vi "ASIC_THx MITAD RANGO.vi"(7 "Espera acceso USB":u32, 8 "error in":errorcluster, 10 "Canal":u8, 11 "ftHandle_in":u32) -> (0 "error out":errorcluster, 3 "ftHandle_out":u32)   [LabVIEW 2009]
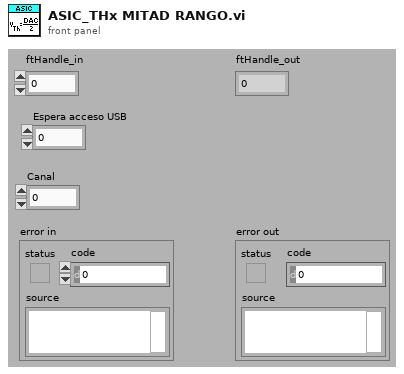
[diagram p1: front panel]
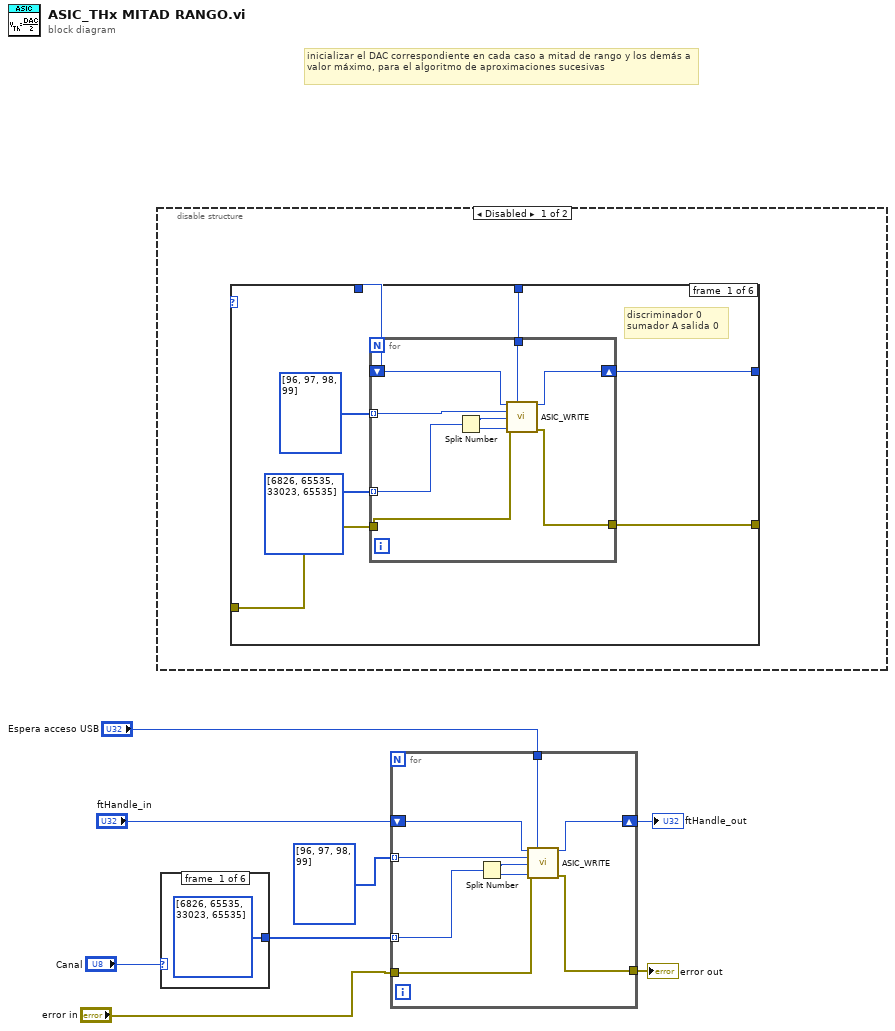
[diagram p0: block diagram]
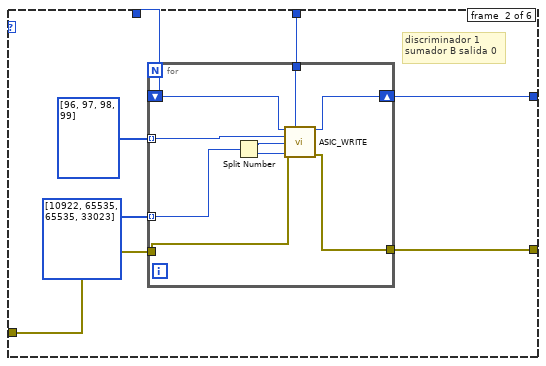
[diagram p2: hidden frame]
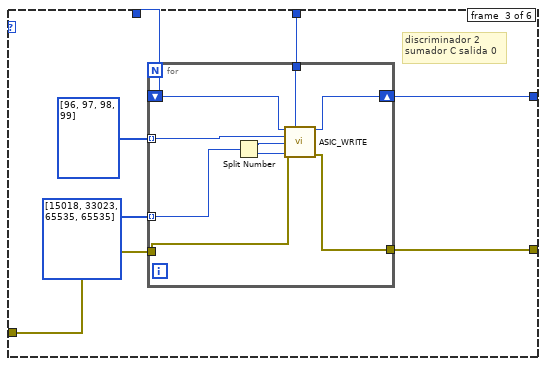
[diagram p3: hidden frame]
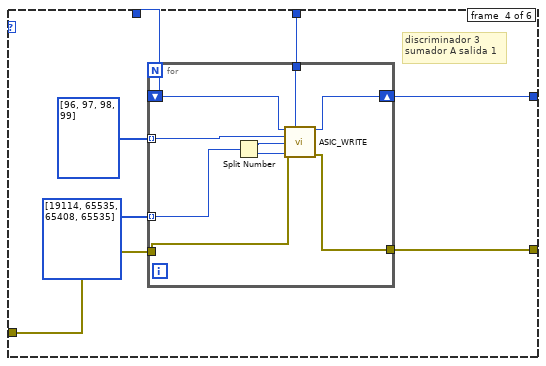
[diagram p4: hidden frame]
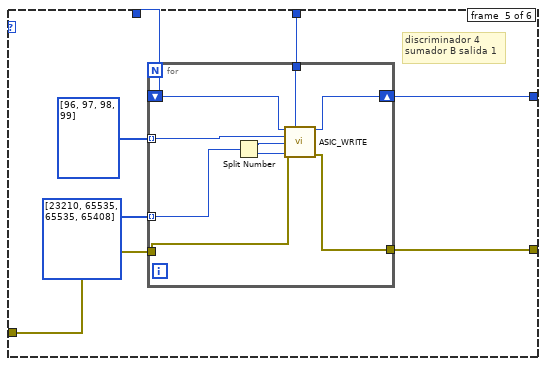
[diagram p5: hidden frame]
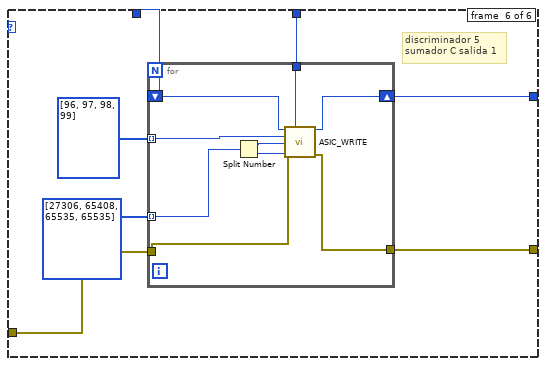
[diagram p6: hidden frame]
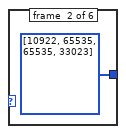
[diagram p8: hidden frame]
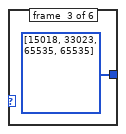
[diagram p9: hidden frame]
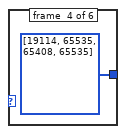
[diagram p10: hidden frame]
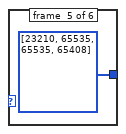
[diagram p11: hidden frame]
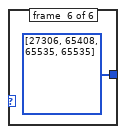
[diagram p12: hidden frame]
diagram:
  # "inicializar el DAC correspondiente en cada caso a mitad de rango y los demás a valor máximo, para el algoritmo de aproximaciones sucesivas"
  n1 = disable-structure shown="Disabled" {
    frame #0 {
      n2 = case shown="5.." {
        tunnel: [w15 w31 w47 w63 w79 w95] -> w10
        tunnel: _ -> [w14 w30 w46 w62 w78 w94]
        tunnel: [w13 w29 w45 w61 w77 w93] -> _
        tunnel: [w12 w27 w44 w60 w76 w92] -> _
        tunnel: [w11 w28 w43 w59 w75 w91] -> w9
        selector: _ -> [_ _ _ _ _ _]
        frame #0 {
          # "discriminador 0\nsumador A salida 0"
          n3 = for {
            shift-right: [w25] -> w12
            shift-left: w15 -> [w26]
            tunnel: i32[] [96, 97, 98, 99] -> [w24] mode=indexing
            tunnel: u16[] [6826, 65535, 33023, 65535] -> [w18] mode=indexing
            tunnel: w14 -> [w23]
            tunnel: [w22] -> w13
            tunnel: w11 -> [w21]
            n4 = Split Number(x=w18) -> (hi(x)=w20:u8, lo(x)=w19:u8)
            n5 = call "ASIC_WRITE.vi"("ftHandle_in"=w26, "Espera acceso USB"=w21, "Direccion Registro Asic"=w24, "Byte Alto"=w20, "Byte Bajo"=w19, "error in"=w23) -> ("ftHandle_out"=w25:u32, "error out"=w22:errorcluster)  [unwired: 8 in]
          }
        }
        frame #1 {
          # "discriminador 1\nsumador B salida 0"
          n6 = for {
            shift-right: [w41] -> w27
            shift-left: w31 -> [w42]
            tunnel: i32[] [96, 97, 98, 99] -> [w40] mode=indexing
            tunnel: u16[] [10922, 65535, 65535, 33023] -> [w34] mode=indexing
            tunnel: w30 -> [w39]
            tunnel: [w38] -> w29
            tunnel: w28 -> [w37]
            n7 = Split Number(x=w34) -> (hi(x)=w36:u8, lo(x)=w35:u8)
            n8 = call "ASIC_WRITE.vi"("ftHandle_in"=w42, "Espera acceso USB"=w37, "Direccion Registro Asic"=w40, "Byte Alto"=w36, "Byte Bajo"=w35, "error in"=w39) -> ("ftHandle_out"=w41:u32, "error out"=w38:errorcluster)  [unwired: 8 in]
          }
        }
        frame #2 {
          # "discriminador 2\nsumador C salida 0"
          n9 = for {
            shift-right: [w57] -> w44
            shift-left: w47 -> [w58]
            tunnel: i32[] [96, 97, 98, 99] -> [w56] mode=indexing
            tunnel: u16[] [15018, 33023, 65535, 65535] -> [w50] mode=indexing
            tunnel: w46 -> [w55]
            tunnel: [w54] -> w45
            tunnel: w43 -> [w53]
            n10 = Split Number(x=w50) -> (hi(x)=w52:u8, lo(x)=w51:u8)
            n11 = call "ASIC_WRITE.vi"("ftHandle_in"=w58, "Espera acceso USB"=w53, "Direccion Registro Asic"=w56, "Byte Alto"=w52, "Byte Bajo"=w51, "error in"=w55) -> ("ftHandle_out"=w57:u32, "error out"=w54:errorcluster)  [unwired: 8 in]
          }
        }
        frame #3 {
          # "discriminador 3\nsumador A salida 1"
          n12 = for {
            shift-right: [w73] -> w60
            shift-left: w63 -> [w74]
            tunnel: i32[] [96, 97, 98, 99] -> [w72] mode=indexing
            tunnel: u16[] [19114, 65535, 65408, 65535] -> [w66] mode=indexing
            tunnel: w62 -> [w71]
            tunnel: [w70] -> w61
            tunnel: w59 -> [w69]
            n13 = Split Number(x=w66) -> (hi(x)=w68:u8, lo(x)=w67:u8)
            n14 = call "ASIC_WRITE.vi"("ftHandle_in"=w74, "Espera acceso USB"=w69, "Direccion Registro Asic"=w72, "Byte Alto"=w68, "Byte Bajo"=w67, "error in"=w71) -> ("ftHandle_out"=w73:u32, "error out"=w70:errorcluster)  [unwired: 8 in]
          }
        }
        frame #4 {
          # "discriminador 4\nsumador B salida 1"
          n15 = for {
            shift-right: [w89] -> w76
            shift-left: w79 -> [w90]
            tunnel: i32[] [96, 97, 98, 99] -> [w88] mode=indexing
            tunnel: u16[] [23210, 65535, 65535, 65408] -> [w82] mode=indexing
            tunnel: w78 -> [w87]
            tunnel: [w86] -> w77
            tunnel: w75 -> [w85]
            n16 = Split Number(x=w82) -> (hi(x)=w84:u8, lo(x)=w83:u8)
            n17 = call "ASIC_WRITE.vi"("ftHandle_in"=w90, "Espera acceso USB"=w85, "Direccion Registro Asic"=w88, "Byte Alto"=w84, "Byte Bajo"=w83, "error in"=w87) -> ("ftHandle_out"=w89:u32, "error out"=w86:errorcluster)  [unwired: 8 in]
          }
        }
        frame #5 {
          # "discriminador 5\nsumador C salida 1"
          n18 = for {
            shift-right: [w105] -> w92
            shift-left: w95 -> [w106]
            tunnel: i32[] [96, 97, 98, 99] -> [w104] mode=indexing
            tunnel: u16[] [27306, 65408, 65535, 65535] -> [w98] mode=indexing
            tunnel: w94 -> [w103]
            tunnel: [w102] -> w93
            tunnel: w91 -> [w101]
            n19 = Split Number(x=w98) -> (hi(x)=w100:u8, lo(x)=w99:u8)
            n20 = call "ASIC_WRITE.vi"("ftHandle_in"=w106, "Espera acceso USB"=w101, "Direccion Registro Asic"=w104, "Byte Alto"=w100, "Byte Bajo"=w99, "error in"=w103) -> ("ftHandle_out"=w105:u32, "error out"=w102:errorcluster)  [unwired: 8 in]
          }
        }
      }
    }
    frame #1 {
    }
  }
  n21 = case shown="0, Default" "Canal" {
    tunnel: [u16[] [6826, 65535, 33023, 65535] u16[] [10922, 65535, 65535, 33023] u16[] [15018, 33023, 65535, 65535] u16[] [19114, 65535, 65408, 65535] u16[] [23210, 65535, 65535, 65408] u16[] [27306, 65408, 65535, 65535]] -> w6
    frame #0 {
    }
    frame #1 {
    }
    frame #2 {
    }
    frame #3 {
    }
    frame #4 {
    }
    frame #5 {
    }
  }
  n22 = for {
    shift-right: [w120] -> w2
    shift-left: "ftHandle_in" -> [w121]
    tunnel: u8[] [96, 97, 98, 99] -> [w119] mode=indexing
    tunnel: w6 -> [w113] mode=indexing
    tunnel: "error in" -> [w118]
    tunnel: [w117] -> w5
    tunnel: "Espera acceso USB" -> [w116]
    n23 = Split Number(x=w113) -> (hi(x)=w115:u8, lo(x)=w114:u8)
    n24 = call "ASIC_WRITE.vi"("ftHandle_in"=w121, "Espera acceso USB"=w116, "Direccion Registro Asic"=w119, "Byte Alto"=w115, "Byte Bajo"=w114, "error in"=w118) -> ("ftHandle_out"=w120:u32, "error out"=w117:errorcluster)  [unwired: 8 in]
  }
  "error out" <- w5
  "ftHandle_out" <- w2
